vi "Run.vi"(6 "Type Y":T2(ring), 7 "Type X":T2(ring), 8 "error in (no error)":errorcluster caption="entrée d'erreur (pas d'erreur)", 9 "Y":string[][](array[string]), 10 "X":string[][](array[string]), 11 "Cosine_similarity.lvclass":refnum<class "Cosine_similarity.lvclass">) -> (0 "error out":errorcluster caption="sortie d'erreur", 2 "Data":T1, 3 "Cosine_similarity.lvclass":refnum<class "Cosine_similarity.lvclass">)   [LabVIEW 2020, in "Cosine_similarity.lvclass"]
doc: "Returns : \n\n- kernel matrix : array\nAn array with shape (n_samples_X, n_samples_Y)."
uses:
  Cosine_similarity.lvclass
  Cosine_similarity.lvclass/Cosine_similarity.ctl
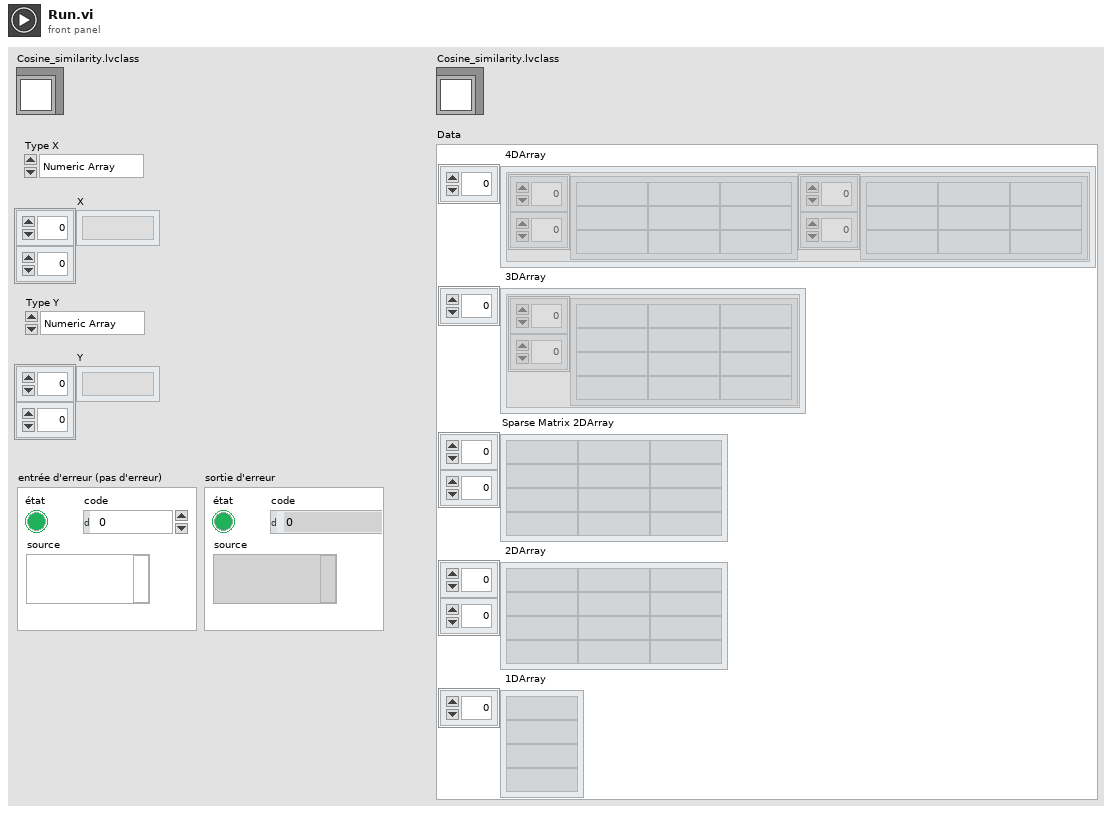
[diagram p1: front panel]
types:
  T1 = cluster{" 4DArray":cluster{"1":string[][], "2":string[][]}[], " 3DArray":cluster{"Tableau":string[][]}[], "Sparse Matrix 2DArray":string[][], " 2DArray":string[][], " 1DArray":string[]}
  T2 = enum16{"Numeric Array", "String Array", "Sparse"}
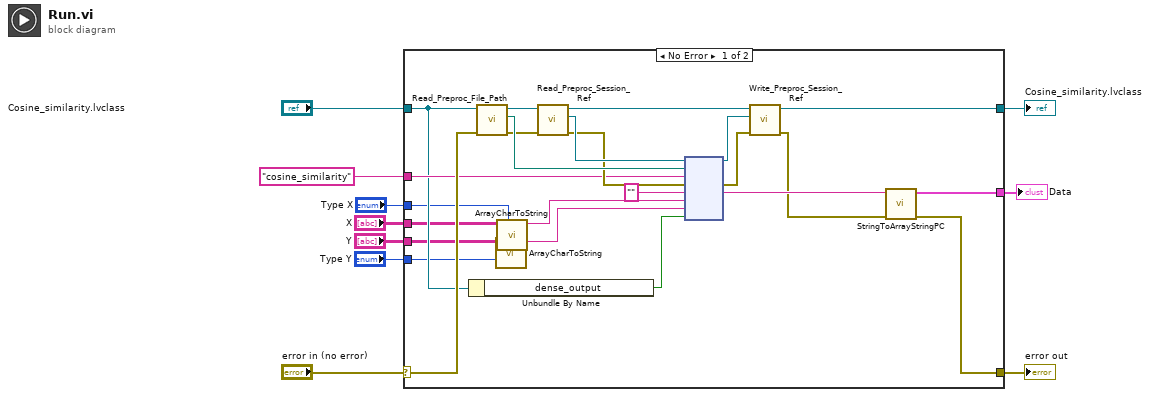
[diagram p0: block diagram]
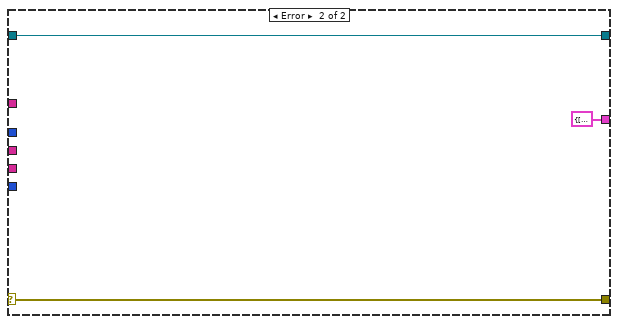
[diagram p2: hidden frame]
diagram:
  n1 = case shown="No Error" "error in (no error)" {
    selector: "error in (no error)" -> [w25 w37]
    tunnel: [w12 w37] -> w9
    tunnel: [w15 w36] -> w7
    tunnel: "Cosine_similarity.lvclass" -> [w23 w36]
    tunnel: "cosine_similarity" ("Fonction") -> [w24 _]
    tunnel: "X" -> [w21 _]
    tunnel: "Y" -> [w20 _]
    tunnel: "Type X" -> [w17 _]
    tunnel: "Type Y" -> [w16 _]
    tunnel: [w11 T1 {" 4DArray"=[], " 3DArray"=[], "Sparse Matrix 2DArray"=[], " 2DArray"=[], " 1DArray"=[]} ("Data")] -> w1
    frame No Error {
      n2 = Unbundle By Name(w23) -> ("dense_output"=w22:bool)
      n3 = call-dynamic "Read_Preproc_File_Path.vi"("error in (no error)"=w25, "Python in"=w23) -> ("error out"=w29:errorcluster, "File_Path"=w32:path, "Python out"=w34:refnum<class "Cosine_similarity.lvclass">)  [unwired: 7 in]
      n4 = call "ArrayCharToString.vi"("Type"=w16, "TAB"=w20) -> ("Instruction"=w18:string)  [unwired: 9 in]
      n5 = call "ArrayCharToString.vi"("Type"=w17, "TAB"=w21) -> ("Instruction"=w19:string)  [unwired: 9 in]
      n6 = call-dynamic "Read_Preproc_Session_Ref.vi"("error in (no error)"=w29, "Python in"=w34) -> ("error out"=w30:errorcluster, "Session_ref"=w31:refnum<k35>, "Python out"=w33:refnum<class "Cosine_similarity.lvclass">)  [unwired: 7 in]
      n7 = node(w31, w32, w24, w30, "", w19, w18, w22) -> (w26:refnum<k35>, w28:errorcluster, w14:string)  [unwired: 3 in, 2 out]
      n8 = call-dynamic "Write_Preproc_Session_Ref.vi"("error in (no error)"=w28, "Session_ref"=w26, "Python in"=w33) -> ("error out"=w13:errorcluster, "Python out"=w15:refnum<class "Cosine_similarity.lvclass">)  [unwired: 7 in]
      n9 = call "StringToArrayStringPC.vi"("sortie d'erreur"=w13, "Return value"=w14) -> ("sortie d'erreur"=w12:errorcluster, "Data"=w11:T1)  [unwired: 8 in]
    }
    frame Error {
    }
  }
  "error out" <- w9
  "Cosine_similarity.lvclass" <- w7
  "Data" <- w1
